vi "get_acq_number.vi"(8 "error in (no error)":errorcluster) -> (0 "error out":errorcluster, 1 "# of acq":i32, 2 "# of meas cycles":i32, 3 "VISA resource name out":refnum<visa-resource-name>)   [LabVIEW 2011]
doc: "returns the number of meas cycle calculate based on the number of acq. divided by the number of frames"
uses:
  global.vi
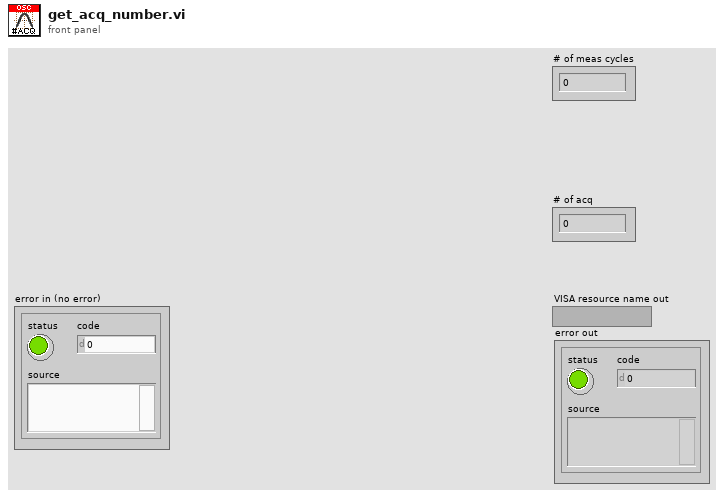
[diagram p1: front panel]
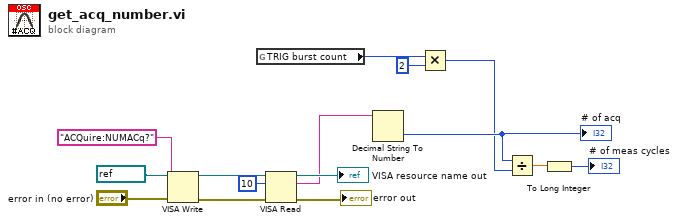
[diagram p0: block diagram]
diagram:
  n1 = VISA Write(VISA resource name=refnum<visa-resource-name> "OSC", write buffer="ACQuire:NUMACq?", error in (no error)="error in (no error)") -> (VISA resource name out=w13:refnum<visa-resource-name>, error out=w9:errorcluster)  [unwired: 1 out]
  n2 = global read "global.vi" "TRIG burst count"() -> (w3:i32)
  n3 = VISA Read(VISA resource name=w13, byte count=u32 10, error in (no error)=w9) -> (VISA resource name out=→"VISA resource name out":refnum<visa-resource-name>, read buffer=w7:string, error out=→"error out":errorcluster)  [unwired: 1 out]
  n4 = Decimal String To Number(string=w7) -> (number=w6:i32)  [unwired: 2 in, 1 out]
  "# of acq" <- w6
  n5 = Multiply(x=w3, y=2) -> (x*y=w1:i32)
  n6 = Divide(x=w6, y=w1) -> (x/y=w5:dbl)
  n7 = To Long Integer(number=w5) -> (32bit integer=→"# of meas cycles":i32)
